vi "0037-Sub_meas.vi"(7 "温湿度データ":dbl[][](array[numeric]), 8 "エラー入力（エラーなし）":errorcluster, 9 "ブール配列":bool[](array[boolean])=[TRUE, TRUE, TRUE, TRUE, TRUE, TRUE, TRUE, FALSE], 11 "device":T1) -> (0 "エラー出力":errorcluster, 3 "deviceOut":T1, 5 "温湿度データ 2":dbl[][](array[numeric]))   [LabVIEW 2014]
uses:
  0034_CP2112-SHT31/LVProject/private/CP2112_device.ctl
panel:
  out "配列 2":dbl[](array[numeric])
  out "配列":dbl[](array[numeric])
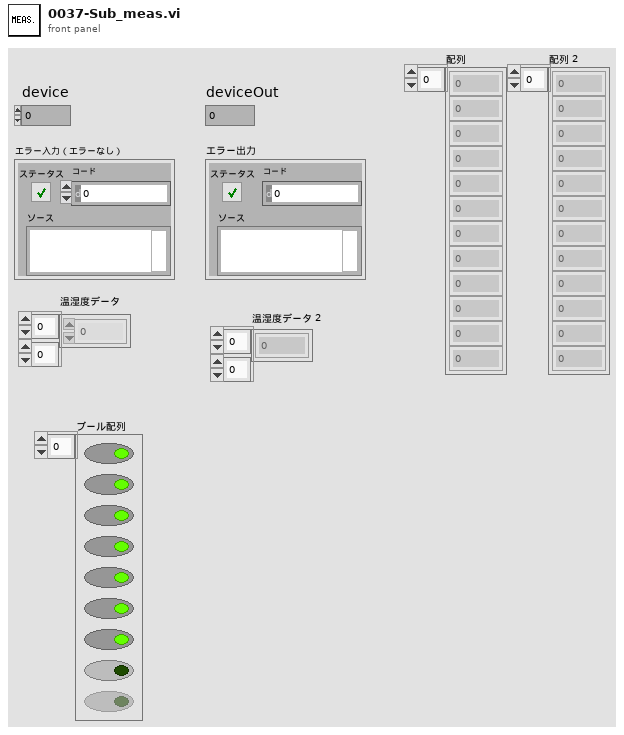
[diagram p1: front panel]
types:
  T1 = typedef "CP2112_device.ctl" = i32
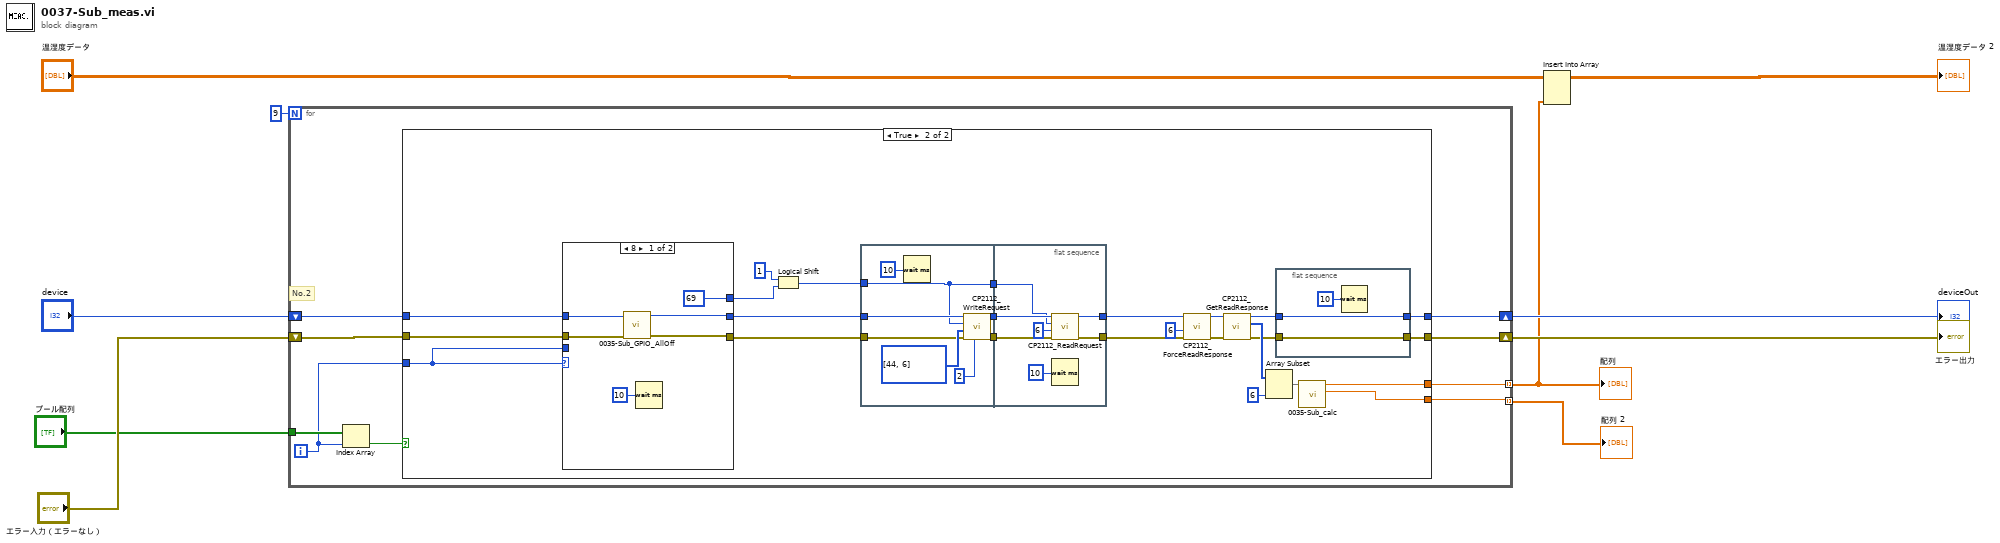
[diagram p0: block diagram]
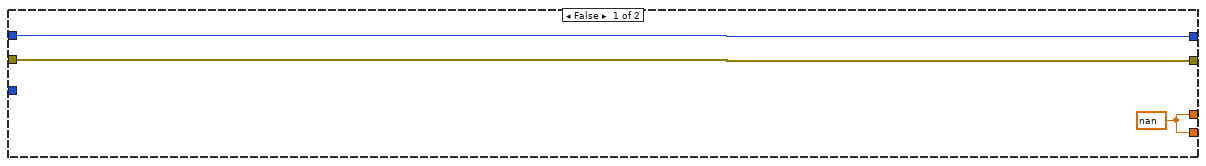
[diagram p2: hidden frame]
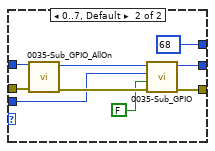
[diagram p3: hidden frame]
diagram:
  n1 = for {
    N: 9 -> [_]
    tunnel: "ブール配列" -> [w15]
    shift-right: [w18] -> w9
    shift-left: "device" -> [w17]
    shift-right: [w19] -> w10
    shift-left: "エラー入力（エラーなし）" -> [w16]
    tunnel: [w12] -> w1 mode=indexing
    tunnel: [w11] -> w2 mode=indexing
    i -> [w13]
    # "No.2"
    n2 = Index Array(array=w15, index=w13) -> (element=w14:bool)
    n3 = case shown="TRUE" w14 {
      tunnel: [w21 w24] -> w19
      tunnel: [w22 w26] -> w18
      tunnel: w17 -> [w22 w42]
      tunnel: w16 -> [w21 w41]
      tunnel: w13 -> [_ w39]
      tunnel: [w20 w38] -> w12
      tunnel: [w20 w37] -> w11
      frame False {
        w20 = nan ("新規要素/部分配列")
      }
      frame True {
        n4 = case shown="8" w39 {
          tunnel: [w68 w80] -> w32
          tunnel: [w67 w79] -> w33
          tunnel: [u32 69 ("ミリ秒待機時間") u32 68 ("ミリ秒待機時間")] -> w35
          tunnel: w42 -> [w70 w77]
          tunnel: w41 -> [w69 w75]
          tunnel: w39 -> [_ w72]
          frame 8 {
            n5 = call "0035-Sub_GPIO_AllOff.vi"("エラー出力 2"=w69, "device"=w70) -> ("エラー出力"=w68:errorcluster, "deviceOut"=w67:T1)  [unwired: 8 in]
            n6 = Wait (ms)(milliseconds to wait=u32 10 ("ミリ秒待機時間")) -> ()  [unwired: 1 out]
          }
          frame 0..7, Default {
            n7 = call "0035-Sub_GPIO_AllOn.vi"("エラー出力 2"=w75, "device"=w77) -> ("エラー出力"=w74:errorcluster, "deviceOut"=w76:T1)  [unwired: 8 in]
            n8 = call "0035-Sub_GPIO.vi"("エラー出力 2"=w74, "ブール"=FALSE, "GPIO"=w72, "device"=w76) -> ("エラー出力"=w80:errorcluster, "deviceOut"=w79:T1)  [unwired: 6 in]
          }
        }
        n9 = Logical Shift(y=1, x=w35) -> (x << y=w34:u32)
        n10 = flat-sequence {
          tunnel: w34 -> [w52]
          tunnel: w33 -> [w54]
          tunnel: w32 -> [w53]
          tunnel: [w58] -> w31
          tunnel: [w57] -> w30
          tunnel: [w52] -> w27
          tunnel: w31 -> [w60]
          tunnel: w30 -> [w62]
          tunnel: [w64] -> w29
          tunnel: [w63] -> w28
          tunnel: w27 -> [w61]
          frame #0 {
            n11 = Wait (ms)(milliseconds to wait=u32 10 ("ミリ秒待機時間")) -> ()  [unwired: 1 out]
            n12 = call "CP2112_WriteRequest.vi"("numBytesToWrite"=i16 2 ("numByteToRead"), "error in (no error)"=w53, "buffer"=u8[] [44, 6], "slaveAddress"=w52, "device"=w54) -> ("error out"=w58:errorcluster, "deviceOut"=w57:T1)  [unwired: 4 in, 1 out]
          }
          frame #1 {
            n13 = call "CP2112_ReadRequest.vi"("error in (no error)"=w60, "numByteToRead"=i16 6, "slaveAddress"=w61, "device"=w62) -> ("error out"=w64:errorcluster, "deviceOut"=w63:T1)  [unwired: 5 in, 1 out]
            n14 = Wait (ms)(milliseconds to wait=u32 10 ("ミリ秒待機時間")) -> ()  [unwired: 1 out]
          }
        }
        n15 = call "CP2112_ForceReadResponse.vi"("error in (no error)"=w29, "numByteToRead"=i16 6, "device"=w28) -> ("error out"=w43:errorcluster, "deviceOut"=w44:T1)  [unwired: 6 in, 1 out]
        n16 = call "CP2112_GetReadResponse.vi"("error in (no error)"=w43, "device"=w44) -> ("error out"=w23:errorcluster, "buffer"=w47:u8[], "deviceOut"=w25:T1)  [unwired: 4 in, 3 out]
        n17 = Array Subset(array=w47, length=6 ("長さ")) -> (w45:u8[])  [unwired: 1 in]
        n18 = flat-sequence {
          tunnel: [w50] -> w26
          tunnel: w25 -> [w50]
          tunnel: [w49] -> w24
          tunnel: w23 -> [w49]
          frame #0 {
            n19 = Wait (ms)(milliseconds to wait=u32 10 ("ミリ秒待機時間")) -> ()  [unwired: 1 out]
          }
        }
        n20 = call "0035-Sub_calc.vi"("Data"=w45) -> ("相対湿度"=w37:dbl, "温度"=w38:dbl)  [unwired: 9 in]
      }
    }
  }
  "エラー出力" <- w10
  "deviceOut" <- w9
  "配列" <- w1
  "配列 2" <- w2
  n21 = Insert Into Array(array="温湿度データ", new element=w1) -> (→"温湿度データ 2":dbl[][])  [unwired: 2 in]
